vi "getElementText.vi"(8 "error in (no error)":errorcluster, 11 "xwpfParagraph in":refnum<class "xwpfParagraph.lvclass">) -> (0 "error out":errorcluster, 2 "Element.Text":string, 3 "xwpfParagraph out":refnum<class "xwpfParagraph.lvclass">)   [LabVIEW 2017, in "Word_Specific.lvlib" / "xwpfParagraph.lvclass"]
uses:
  xwpfParagraph.lvclass
  Get Runs.Text.vi
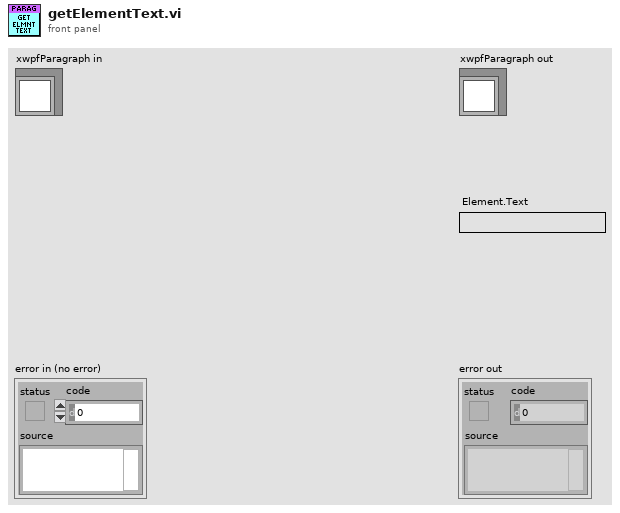
[diagram p1: front panel]
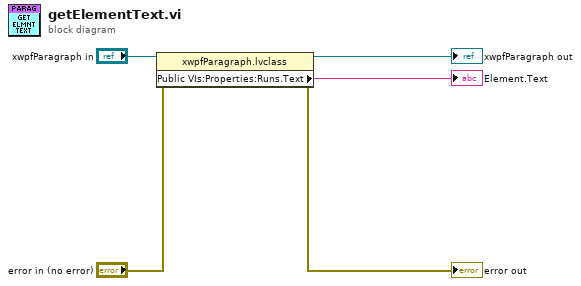
[diagram p0: block diagram]
diagram:
  n1 = property class="xwpfParagraph.lvclass"(reference="xwpfParagraph in", error in="error in (no error)") -> (reference out=→"xwpfParagraph out":refnum<class "xwpfParagraph.lvclass">, error out=→"error out":errorcluster, "Public VIs:Properties:Runs.Text"=→"Element.Text":string)
